vi "1.4.1-Encoder Math Simple.vi"(1 "B":bool, 2 "A":bool) -> (0 "Numeric":fxp<+/-,2,2>)   [LabVIEW 2010]
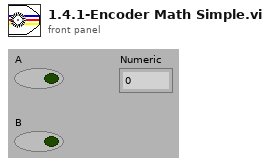
[diagram p1: front panel]
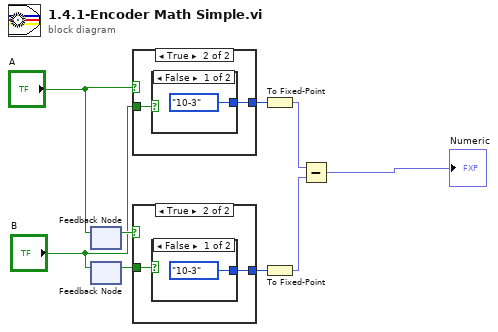
[diagram p0: block diagram]
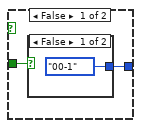
[diagram p2: hidden frame]
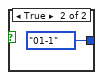
[diagram p3: hidden frame]
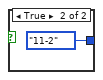
[diagram p4: hidden frame]
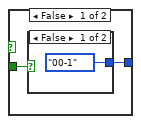
[diagram p5: hidden frame]
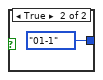
[diagram p6: hidden frame]
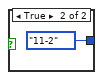
[diagram p7: hidden frame]
diagram:
  n1 = feedback #1() -> (w3:bool)  [unwired: 1 in]
  n2 = feedback-in #1("A") -> ()
  n3 = feedback #2() -> (w4:bool)  [unwired: 1 in]
  n4 = feedback-in #2("B") -> ()
  n5 = case shown="True" "A" {
    tunnel: "B" -> [w11 w15]
    tunnel: [w10 w14] -> w7
    frame False {
      n6 = case shown="False" w11 {
        tunnel: [enum8{"00-1", "01-1", "11-2", "10-3"}."00-1" enum8{"00-1", "01-1", "11-2", "10-3"}."01-1"] -> w10
        frame False {
        }
        frame True {
        }
      }
    }
    frame True {
      n7 = case shown="False" w15 {
        tunnel: [enum8{"00-1", "01-1", "11-2", "10-3"}."10-3" enum8{"00-1", "01-1", "11-2", "10-3"}."11-2"] -> w14
        frame False {
        }
        frame True {
        }
      }
    }
  }
  n8 = case shown="True" w3 {
    tunnel: w4 -> [w19 w23]
    tunnel: [w18 w22] -> w5
    frame False {
      n9 = case shown="False" w19 {
        tunnel: [enum8{"00-1", "01-1", "11-2", "10-3"}."00-1" enum8{"00-1", "01-1", "11-2", "10-3"}."01-1"] -> w18
        frame False {
        }
        frame True {
        }
      }
    }
    frame True {
      n10 = case shown="False" w23 {
        tunnel: [enum8{"00-1", "01-1", "11-2", "10-3"}."10-3" enum8{"00-1", "01-1", "11-2", "10-3"}."11-2"] -> w22
        frame False {
        }
        frame True {
        }
      }
    }
  }
  n11 = To Fixed-Point(number=w7) -> (fixed-point=w8:fxp<+/-,2,2>)  [unwired: 1 in]
  n12 = To Fixed-Point(number=w5) -> (fixed-point=w6:fxp<+/-,2,2>)  [unwired: 1 in]
  n13 = Subtract(x=w8, y=w6) -> (x-y=→"Numeric":fxp<+/-,2,2>)
